vi "Create or update project ini file.vi"(0 "Project file path":path, 5 "Comment":string, 7 "Project information":T1={"Job and Site"={"Project Number"="test", "Client Company"="test", "Country"="test", "Field"="test", "Rig"="Afghanistan", "Well"=""}, "Tool"={"Tractor type"="test", "Tool"="test", "Serial #"="test"}, "Run Information"={"Active Run"=FALSE, "String Check Rec"=FALSE, "Run Number"=0, "Time of File Start"=""}}, 11 "error in (no error)":errorcluster) -> (15 "error out":errorcluster)   [LabVIEW 2011]
uses:
  Project in icluster.ctl
  GUI/Job setup/Job and site cluster.ctl
  emi cndiates/List of all contrys(combo box).ctl
  GUI/Job setup/Tool registration ID.ctl
  Run Information.ctl
  <vilib>/Utility/libraryn.llb/Check if File or Folder Exists.vi
  <vilib>/Utility/VariantDataType/VariantType.lvlib
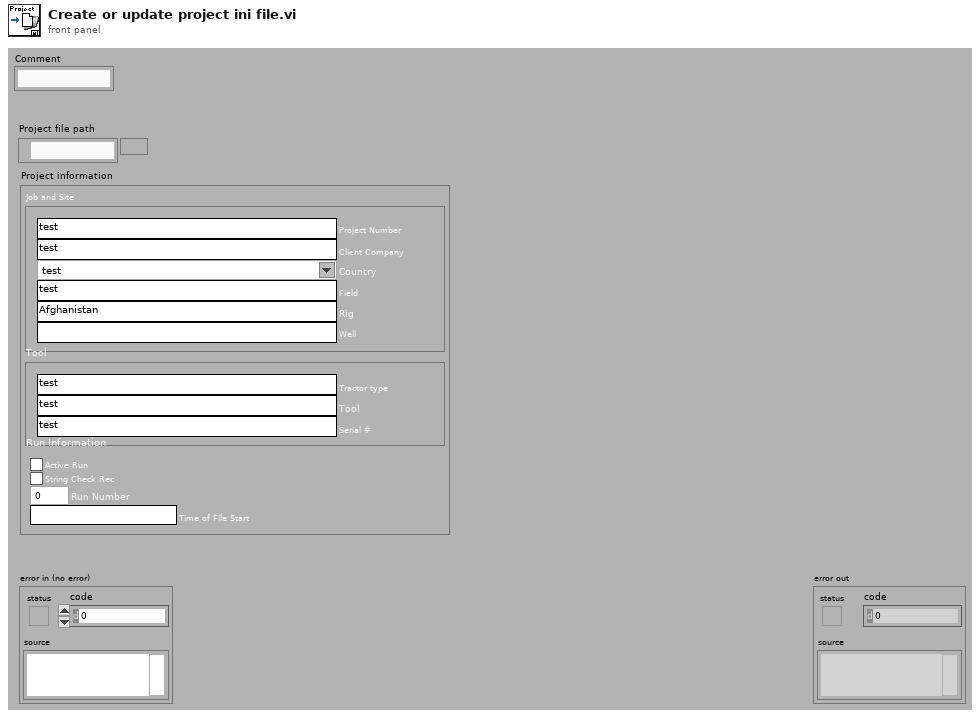
[diagram p1: front panel]
types:
  T1 = typedef "Project in icluster.ctl" = cluster{"Job and Site":T2, "Tool":T4, "Run Information":T5}
  T2 = typedef "Job and site cluster.ctl" = cluster{"Project Number":string, "Client Company":string, "Country":T3, "Field":string, "Rig":string, "Well":string}
  T3 = typedef "List of all contrys(combo box).ctl" = string
  T4 = typedef "Tool registration ID.ctl" = cluster{"Tractor type":string, "Tool":string, "Serial #":string}
  T5 = typedef "Run Information.ctl" = cluster{"Active Run":bool, "String Check Rec":bool, "Run Number":i32, "Time of File Start":string}
  T6 = enum16{"open", "replace", "create", "open or create", "replace or create", "replace or create with confirmation"}
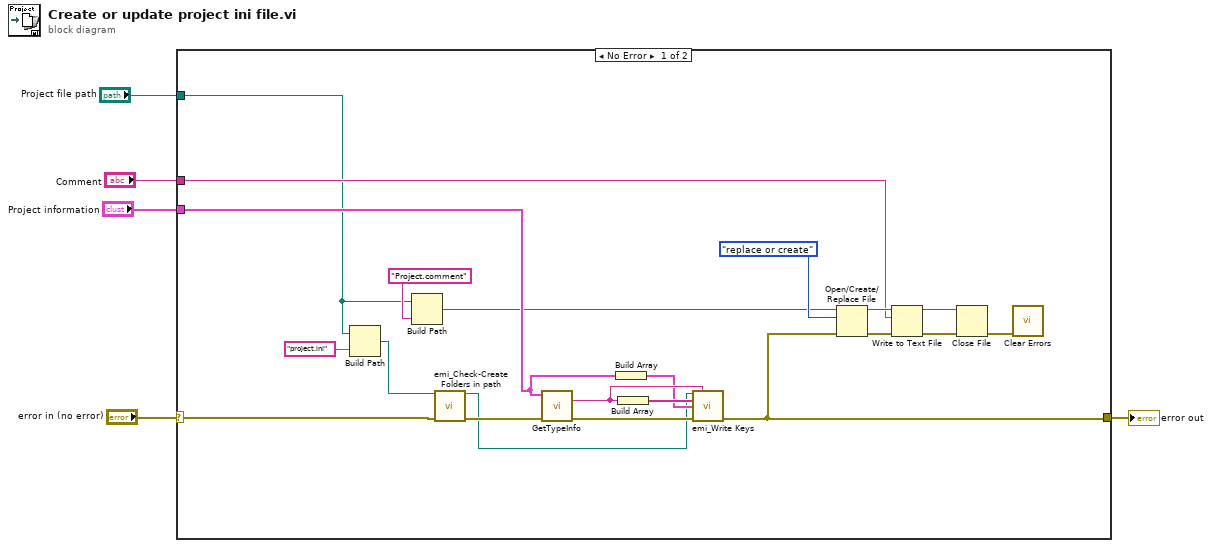
[diagram p0: block diagram]
diagram:
  n1 = case shown="No Error" "error in (no error)" {
    selector: "error in (no error)" -> [w11 w27]
    tunnel: [w15 w27] -> w4
    tunnel: "Project information" -> [w22 _]
    tunnel: "Project file path" -> [w8 _]
    tunnel: "Comment" -> [w14 _]
    frame No Error {
      n2 = Build Path(base path=w8, name or relative path="project.ini") -> (appended path=w12:path)
      n3 = Build Path(base path=w8, name or relative path="Project.comment") -> (appended path=w7:path)
      n4 = call "emi_Check-Create Folders in path.vi"("Path including file"=w12, "error in (no error)"=w11) -> ("Path out"=w6:path, "error out"=w10:errorcluster)  [unwired: 11 in, 1 out]
      n5 = call <vilib>:"GetTypeInfo.vi"("error in (no error)"=w10, "Variant"=w22) -> ("error out"=w24:errorcluster, "Name"=w26:string)  [unwired: 5 in, 3 out]
      n6 = Build Array(w22) -> (w23:T1[])
      n7 = Build Array(w26) -> (w25:string[])
      n8 = call "emi_Write Keys.vi"("Ini Path(..app../config.ini)"=w6, "Section"=w26, "Key Names"=w25, "Values"=w23, "error in (no error)"=w24) -> ("error out"=w15:errorcluster)  [unwired: 9 in, 1 out]
      n9 = Open/Create/Replace File(file path (use dialog)=w7, error in=w15, operation (0:open)=T6."replace or create") -> (refnum out=w19:refnum<file>, error out=w20:errorcluster)  [unwired: 3 in, 1 out]
      n10 = Write to Text File(file (use dialog)=w19, text=w14, error in=w20) -> (refnum out=w17:refnum<file>, error out=w18:errorcluster)  [unwired: 1 in, 1 out]
      n11 = Close File(refnum=w17, error in=w18) -> (error out=w16:errorcluster)  [unwired: 1 out]
      n12 = call <vilib>:"Clear Errors.vi"("error in (no error)"=w16) -> ()  [unwired: 6 in, 1 out]
    }
    frame Error {
    }
  }
  "error out" <- w4
